vi "ELY_estado_analyzer (SubVI).vi"(11 "Numeric":u16) -> (1 "Colors [4]":cluster{u32, u32}[](array[cluster]), 2 "Boolean 2":bool, 3 "Caption.Text":string, 4 "Boolean":bool)   [LabVIEW 2024, in "S7-1200_OPCUA.lvlib"]
uses:
  S7-1200_OPCUA.lvlib
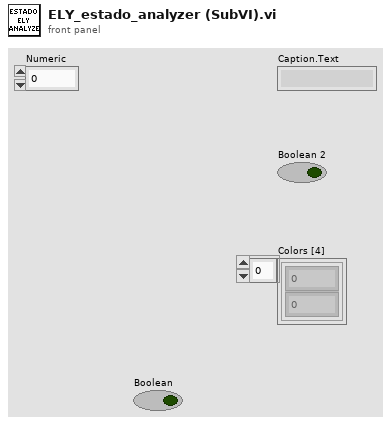
[diagram p1: front panel]
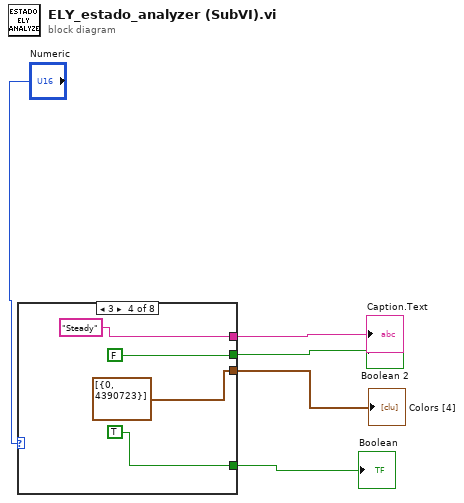
[diagram p0: block diagram]
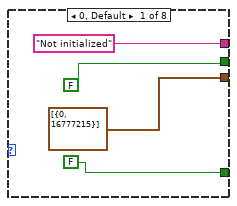
[diagram p2: hidden frame]
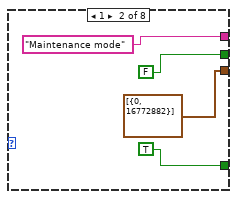
[diagram p3: hidden frame]
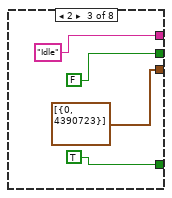
[diagram p4: hidden frame]
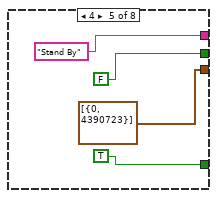
[diagram p5: hidden frame]
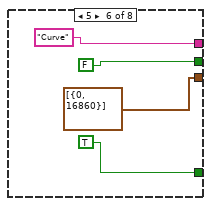
[diagram p6: hidden frame]
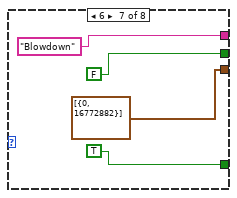
[diagram p7: hidden frame]
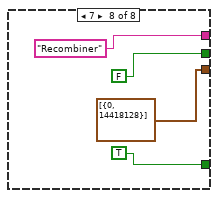
[diagram p8: hidden frame]
diagram:
  n1 = case shown="3" "Numeric" {
    tunnel: [FALSE FALSE FALSE FALSE FALSE FALSE FALSE FALSE] -> w2
    tunnel: [FALSE TRUE TRUE TRUE TRUE TRUE TRUE TRUE] -> w3
    tunnel: [cluster{u32, u32}[] [{0, 16777215}] ("Colors [4]") cluster{u32, u32}[] [{0, 16772882}] ("Colors [4]") cluster{u32, u32}[] [{0, 4390723}] ("Colors [4]") cluster{u32, u32}[] [{0, 4390723}] ("Colors [4]") cluster{u32, u32}[] [{0, 4390723}] ("Colors [4]") cluster{u32, u32}[] [{0, 16860}] ("Colors [4]") cluster{u32, u32}[] [{0, 16772882}] ("Colors [4]") cluster{u32, u32}[] [{0, 14418128}] ("Colors [4]")] -> w4
    tunnel: ["Not initialized" ("Caption.Text") "Maintenance mode" ("Caption.Text") "Idle" ("Caption.Text") "Steady" ("Caption.Text") "Stand By" ("Caption.Text") "Curve" ("Caption.Text") "Blowdown" ("Caption.Text") "Recombiner" ("Caption.Text")] -> w5
    frame 0, Default {
    }
    frame 1 {
    }
    frame 2 {
    }
    frame 3 {
    }
    frame 4 {
    }
    frame 5 {
    }
    frame 6 {
    }
    frame 7 {
    }
  }
  "Caption.Text" <- w5
  "Colors [4]" <- w4
  "Boolean" <- w3
  "Boolean 2" <- w2
